vi "sub-Language-get sid.vi"(0 "str":string) -> (1 "sid":u32 format="%04x", 2 "valid?":bool)   [LabVIEW 2011]
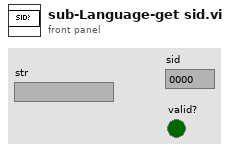
[diagram p1: front panel]
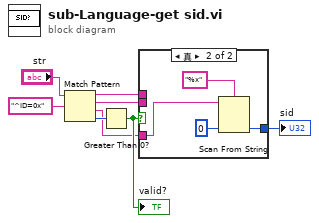
[diagram p0: block diagram]
diagram:
  n1 = Match Pattern(string="str", regular expression="^ID=0x" ("正则表达式")) -> (before substring=w2:string, match substring=w4:string, after substring=w1:string, offset past match=w6:i32)  [unwired: 1 in]
  n2 = Greater Than 0?(x=w6) -> (x > 0?=w5:bool)
  "valid?" <- w5
  n3 = case shown="真" w5 {
    tunnel: w4 -> [_ _]
    tunnel: [_ w10] -> w3
    tunnel: w2 -> [_ _]
    tunnel: w1 -> [_ w9]
    frame False {
    }
    frame True {
      n4 = Scan From String(format string="%x" ("格式字符串"), input string=w9, default 1=u32 0 ("默认值 1")) -> (output 1=w10:u32)  [unwired: 2 in, 3 out]
    }
  }
  "sid" <- w3
